vi "Rebuild Lua filter.vi"   [LabVIEW 2019, in "LINXx.lvlib"]
doc: "Dev helper to automatically generate Lua script for parsing USB serial comms with WireShark"
uses:
  LINXx.lvlib
types:
  T1 = enum16{"Native", "Native Command Line", "UNIX", "Macintosh", "DOS"}
  T2 = enum16{"open", "replace", "create", "open or create", "replace or create", "replace or create with confirmation"}
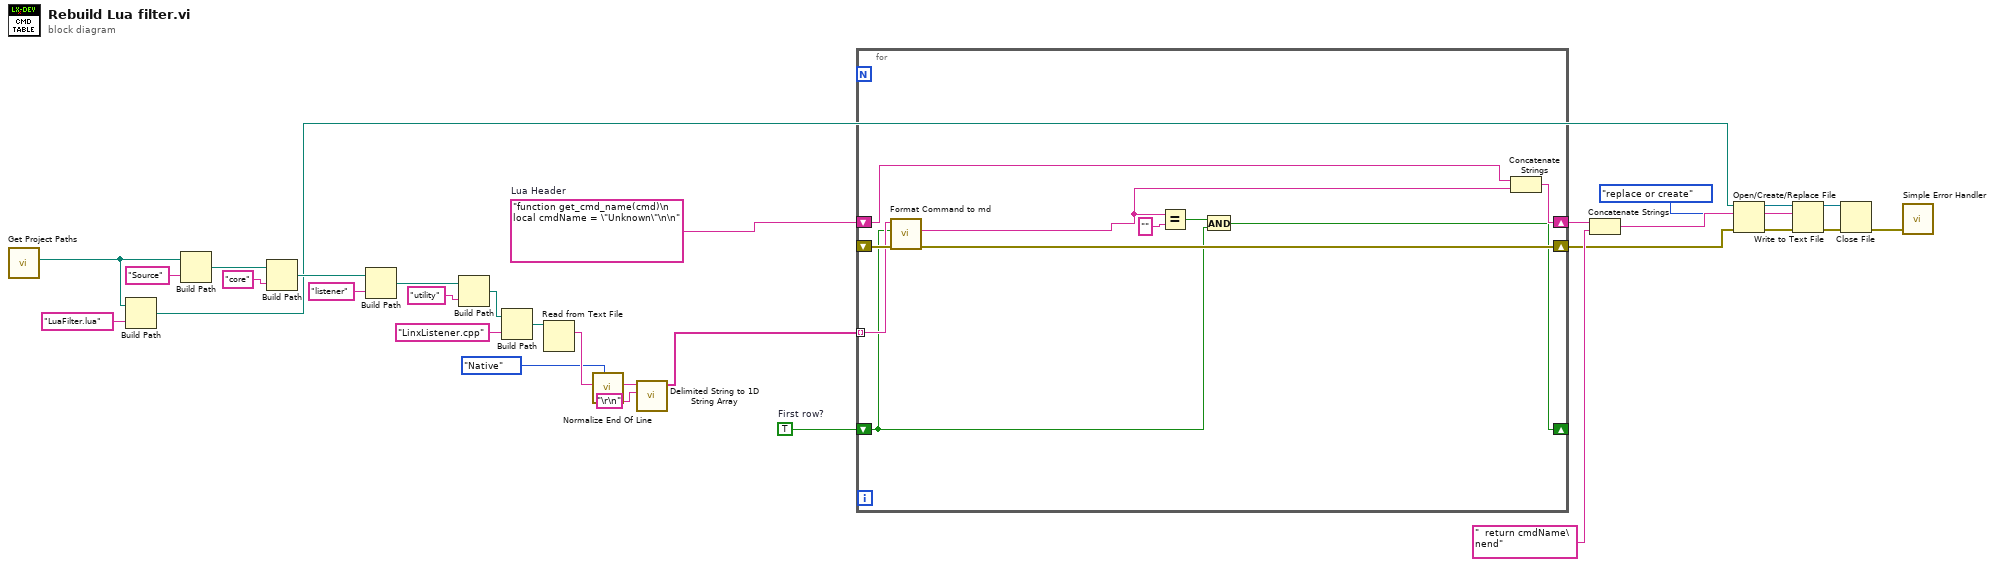
[diagram p0: block diagram]
diagram:
  w17 = TRUE  # First row?
  w18 = "function get_cmd_name(cmd)\n  local cmdName = \"Unknown\"\n\n"  # Lua Header
  n1 = call "Get Project Paths.vi"() -> ("Firmware path"=w19:path)  [unwired: 9 in, 2 out]
  n2 = Build Path(base path=w19, name or relative path="LuaFilter.lua") -> (appended path=w8:path)
  n3 = Build Path(base path=w19, name or relative path="Source") -> (appended path=w28:path)
  n4 = Build Path(base path=w28, name or relative path="core") -> (appended path=w26:path)
  n5 = Build Path(base path=w26, name or relative path="listener") -> (appended path=w24:path)
  n6 = Build Path(base path=w24, name or relative path="utility") -> (appended path=w22:path)
  n7 = Build Path(base path=w22, name or relative path="LinxListener.cpp") -> (appended path=w21:path)
  n8 = Read from Text File(file (use dialog)=w21) -> (text=w5:string)  [unwired: 3 in, 3 out]
  n9 = call <vilib>:"Normalize End Of Line.vi"("end of line (Native)"=T1."Native", "string in"=w5) -> ("string out"=w3:string)  [unwired: 6 in]
  n10 = call <vilib>:"Delimited String to 1D String Array.vi"("delimiter"="\r\n", "delimited string"=w3) -> ("string array"=w4:string[])  [unwired: 9 in]
  n11 = for {
    tunnel: w4 -> [w33] mode=indexing
    shift-right: [w39] -> w14
    shift-left: w18 -> [w40]
    shift-right: [w37] -> w9
    shift-left: _ -> [w38]
    shift-right: [w34] -> _
    shift-left: w17 -> [w31]
    n12 = call "Format Command to md.vi"("error in (no error)"=w38, "firstRow?"=w31, "line"=w33) -> ("error out"=w37:errorcluster, "lua row"=w32:string)  [unwired: 6 in, 1 out]
    n13 = Equal?(x=w32, y="") -> (x = y?=w35:bool)
    n14 = And(x=w35, y=w31) -> (x .and. y?=w34:bool)
    n15 = Concatenate Strings(w40, w32) -> (w39:string)
  }
  n16 = Concatenate Strings(w14, "  return cmdName\nend" ("string")) -> (w13:string)
  n17 = Open/Create/Replace File(file path (use dialog)=w8, error in=w9, operation (0:open)=T2."replace or create") -> (refnum out=w11:refnum<file>, error out=w12:errorcluster)  [unwired: 3 in, 1 out]
  n18 = Write to Text File(file (use dialog)=w11, text=w13, error in=w12) -> (refnum out=w10:refnum<file>, error out=w16:errorcluster)  [unwired: 1 in, 1 out]
  n19 = Close File(refnum=w10, error in=w16) -> (error out=w6:errorcluster)  [unwired: 1 out]
  n20 = call <vilib>:"Simple Error Handler.vi"("error in (no error)"=w6) -> ()  [unwired: 4 in, 5 out]
